vi "scan ready.vi"() -> ()   [LabVIEW 2020, in "Coarse Approach.lvclass"]
uses:
  Coarse Approach.lvclass
  PI P123.01 & PiezoDrive TD250 & NI USB 7855R/PI P123.01 & PiezoDrive TD250 & NI USB 7855R.lvclass
  Newport Model 8742/New Focus Model 8742.lvclass
panel:
  out "Coarse Approach.lvclass":refnum<class "Coarse Approach.lvclass">
  in  "Coarse Approach.lvclass":refnum<class "Coarse Approach.lvclass">
  in  "Numeric":i32
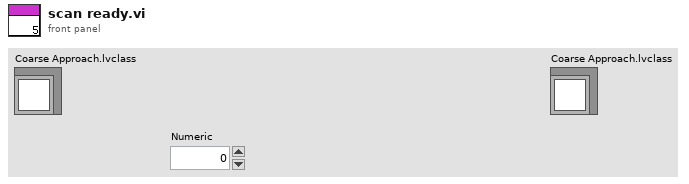
[diagram p1: front panel]
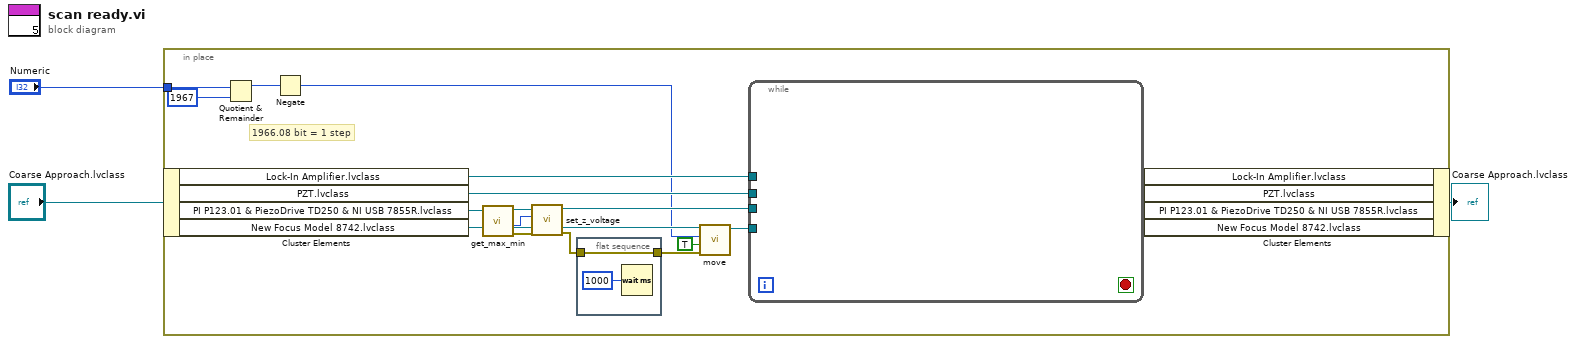
[diagram p0: block diagram]
diagram:
  n1 = in-place {
    in-place-border: "Numeric" -> [w19]
    # "1966.08 bit = 1 step"
    n2 = in-place-cluster #1("Coarse Approach.lvclass") -> ("Lock-In Amplifier.lvclass"=w12:refnum<class "Lock-In Amplifier.lvclass">, "PZT.lvclass"=w11:refnum<class "PZT.lvclass">, "PI P123.01 & PiezoDrive TD250 & NI USB 7855R.lvclass"=w15:refnum<class "PI P123.01 & PiezoDrive TD250 & NI USB 7855R.lvclass">, "New Focus Model 8742.lvclass"=w9:refnum<class "New Focus Model 8742.lvclass">)
    n3 = Quotient & Remainder(x=w19, y=1967) -> (x-y*floor(x/y)=w17:i32)  [unwired: 1 out]
    n4 = Negate(x=w17) -> (-x=w6:i32)
    n5 = call "get_max_min.vi"("PI P123.01 & PiezoDrive TD250 & NI USB 7855R.lvclass"=w15) -> ("error out"=w13:errorcluster, "Piezo_minimum"=w16:i16, "PI P123.01 & PiezoDrive TD250 & NI USB 7855R.lvclass 2"=w14:refnum<class "PI P123.01 & PiezoDrive TD250 & NI USB 7855R.lvclass">)  [unwired: 7 in, 1 out]
    n6 = call "set_z_voltage.vi"("error in (no error)"=w13, "Z Voltage (V)"=w16, "PI P123.01 & PiezoDrive TD250 & NI USB 7855R in"=w14) -> ("error out"=w5:errorcluster, "PI P123.01 & PiezoDrive TD250 & NI USB 7855R out"=w10:refnum<class "PI P123.01 & PiezoDrive TD250 & NI USB 7855R.lvclass">)  [unwired: 7 in]
    n7 = flat-sequence {
      tunnel: w5 -> [w21]
      tunnel: [w21] -> w4
      frame #0 {
        n8 = Wait (ms)(milliseconds to wait=u32 1000) -> ()  [unwired: 1 out]
      }
    }
    n9 = call "move.vi"("error in"=w4, "Relative? (T)"=TRUE, "Destination (steps)"=w6, "Newport Model 8742 in"=w9) -> ("Newport Model 8742 out"=w8:refnum<class "New Focus Model 8742.lvclass">)  [unwired: 6 in, 1 out]
    n10 = while {
      tunnel: w12 -> [_]
      tunnel: w11 -> [_]
      tunnel: w10 -> [_]
      tunnel: w8 -> [_]
      stop <- _ stop-if-true
    }
    n11 = in-place-cluster #1() -> (→"Coarse Approach.lvclass":refnum<class "Coarse Approach.lvclass">)  [unwired: 4 in]
  }
